vi "AOL Z Cal-Get current cal.vi"() -> (1 "FOVs":dbl[](array[numeric]), 3 "Previous cal":dbl[][](array[numeric]))   [LabVIEW 2013]
uses:
  Typedefs/Functional global standard states.ctl
panel:
  out "Number of FOV":i32
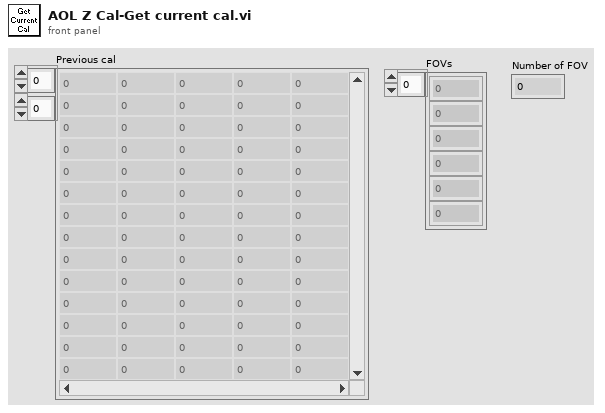
[diagram p1: front panel]
types:
  T1 = typedef "Functional global standard states.ctl" = enum16{"Initialise", "Read", "Write", "Load", "Save", "Clear"}
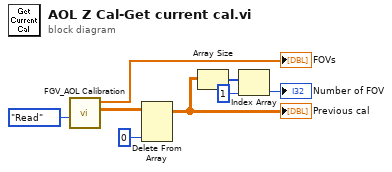
[diagram p0: block diagram]
diagram:
  n1 = call "FGV_AOL Calibration.vi"("Function"=Functional_global_standard_states."Read") -> ("Calibration Data"=w7:dbl[][], "FOV values"=→"FOVs":dbl[])  [unwired: 8 in, 1 out]
  n2 = Delete From Array(array=w7, index (col)=0 ("disabled index (col)")) -> (array with subset deleted=w1:dbl[][])  [unwired: 2 in, 1 out]
  "Previous cal" <- w1
  n3 = Array Size(array=w1) -> (size(s)=w5:i32[])
  n4 = Index Array(array=w5, index=1) -> (element=→"Number of FOV":i32)
